vi "TCPCOMUNICACION.vi"() -> ()   [LabVIEW 2017]
panel:
  out "Slide 2":dbl(slide) scale=0.0..300.0
  out "Slide":dbl(slide) scale=0.0..300.0
  in  "stop 2":bool
  out "Numeric 5":dbl
  out "Numeric 6":dbl
  out "Datos recibidos vía TCP":cluster{dbl, dbl}(graph)
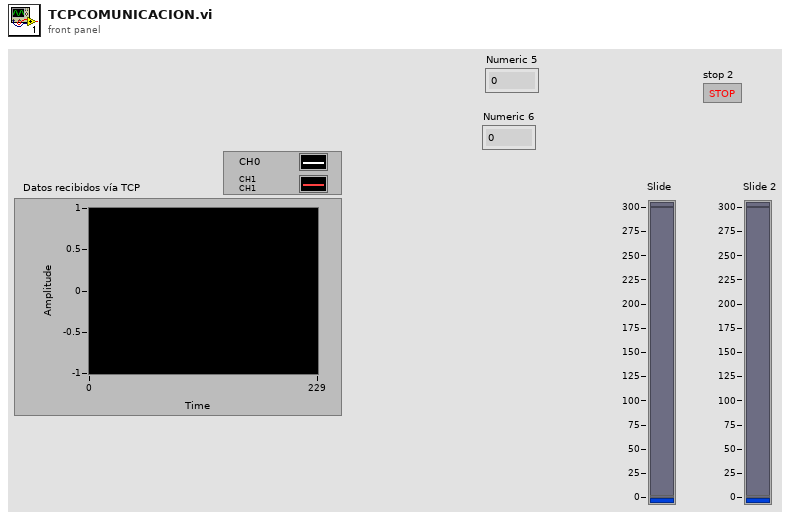
[diagram p1: front panel]
types:
  T1 = enum16{"Standard", "Buffered", "CRLF", "Immediate"}
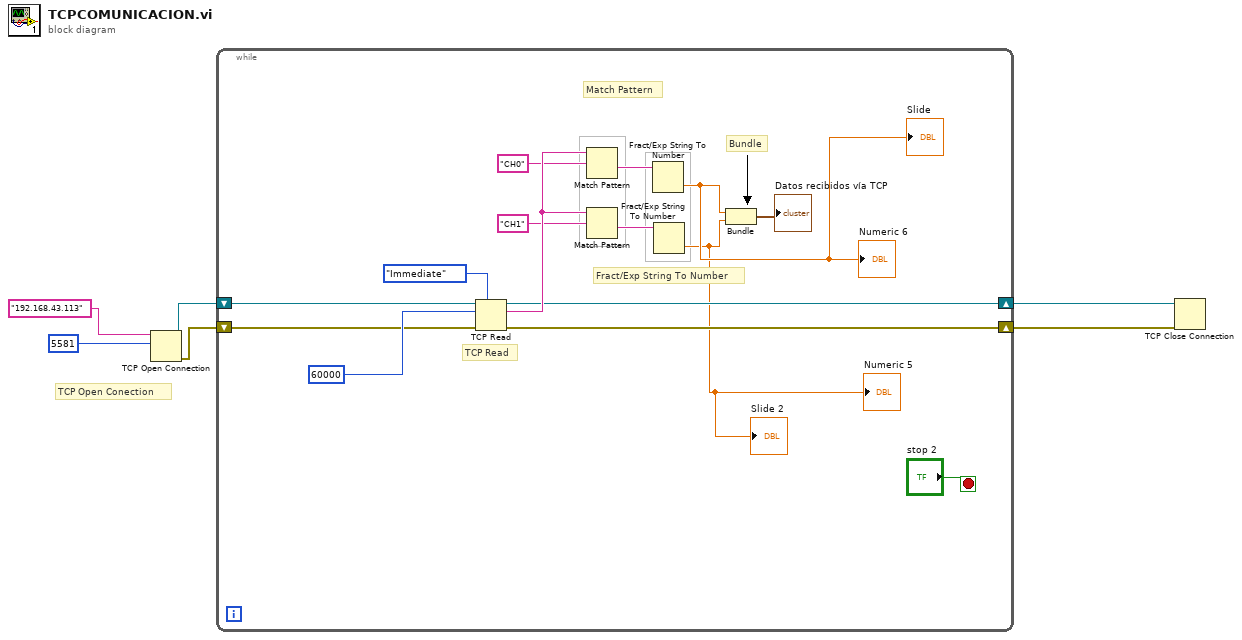
[diagram p0: block diagram]
diagram:
  # "TCP Open Conection"
  n1 = TCP Open Connection(address="192.168.43.113", remote port or service name=u16 5581) -> (connection ID=w3:refnum<k5>, error out=w4:errorcluster)  [unwired: 3 in]
  n2 = while {
    shift-right: [w11] -> w2
    shift-left: w4 -> [w13]
    shift-right: [w10] -> w1
    shift-left: w3 -> [w12]
    stop <- "stop 2" stop-if-true
    # "Bundle"
    # "TCP Read"
    # "Fract/Exp String To Number"
    # "Match Pattern"
    n3 = TCP Read(connection ID=w12, bytes to read=60000, error in (no error)=w13, 7:T1."Immediate" ("mode (standard)")) -> (connection ID out=w10:refnum<k5>, data out=w20:string, error out=w11:errorcluster)  [unwired: 1 in]
    n4 = Match Pattern(string=w20, regular expression="CH0") -> (after substring=w17:string)  [unwired: 1 in, 3 out]
    n5 = Match Pattern(string=w20, regular expression="CH1") -> (after substring=w19:string)  [unwired: 1 in, 3 out]
    n6 = Fract/Exp String To Number(string=w17) -> (number=w8:dbl)  [unwired: 3 in, 1 out]
    "Numeric 6" <- w8
    "Slide" <- w8
    n7 = Fract/Exp String To Number(string=w19) -> (number=w7:dbl)  [unwired: 3 in, 1 out]
    "Numeric 5" <- w7
    "Slide 2" <- w7
    n8 = Bundle(w8, w7) -> (→"Datos recibidos vía TCP":cluster{dbl, dbl})  [unwired: 1 in]
  }
  n9 = TCP Close Connection(connection ID=w1, error in (no error)=w2) -> ()  [unwired: 1 in, 2 out]
